vi "TCP-Get Local Address.vi"() -> (8 "net address":u32, 10 "address":string)   [LabVIEW 2020]
uses:
  0742cc26-4acf-47fd-8537-03877dbc5314.vi
  <vilib>/Comparison/Less/Less Functor/Less Functor.lvclass
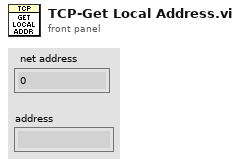
[diagram p1: front panel]
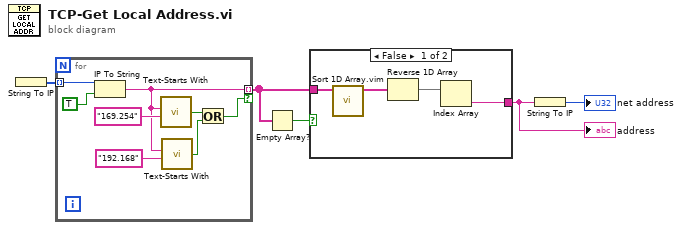
[diagram p0: block diagram]
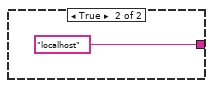
[diagram p2: hidden frame]
diagram:
  n1 = String To IP() -> (0:w1:u32[])  [unwired: 1 in]
  n2 = for {
    tunnel: w1 -> [w12] mode=indexing
    tunnel: [w7] -> w3 mode=indexing if=w8
    n3 = IP To String(1:TRUE ("dot notation? (F)"), 2:w12) -> (0:w7:string)
    n4 = call "Text-Starts With.vi"("Starts with"="169.254", "String"=w7) -> ("result"=w9:bool)  [unwired: 4 in]
    n5 = call "Text-Starts With.vi"("Starts with"="192.168", "String"=w7) -> ("result"=w6:bool)  [unwired: 4 in]
    n6 = Or(x=w9, y=w6) -> (x .or. y?=w8:bool)
  }
  n7 = Empty Array?(array=w3) -> (empty?=w4:bool)
  n8 = case shown="False" w4 {
    tunnel: w3 -> [w16 _]
    tunnel: [w17 "localhost"] -> w5
    frame False {
      n9 = call "Sort 1D Array.vim"("unsorted array"=w16) -> ("sorted array"=w15:string[])  [unwired: 10 in]
      n10 = Reverse 1D Array(array=w15) -> (reversed array=w14:string[])
      n11 = Index Array(array=w14) -> (element=w17:string)  [unwired: 1 in]
    }
    frame True {
    }
  }
  "address" <- w5
  n12 = String To IP(1:w5) -> (0:→"net address":u32)
